vi "ObtenerDatosdelatabla.vi"(7 "tipo_gen":string="externo", 9 "Column":i32, 10 "Row":i32, 11 "Prueba32 in":refnum<class "Prueba031.lvclass">) -> (3 "Prueba32 out":refnum<class "Prueba031.lvclass">)   [LabVIEW 2019, in "Prueba031.lvclass"]
uses:
  Prueba031.lvclass
  Prueba031.lvclass/Prueba031.ctl
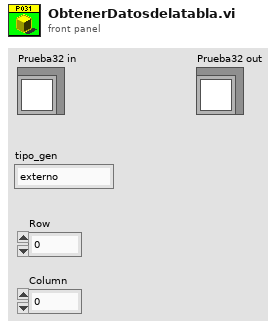
[diagram p1: front panel]
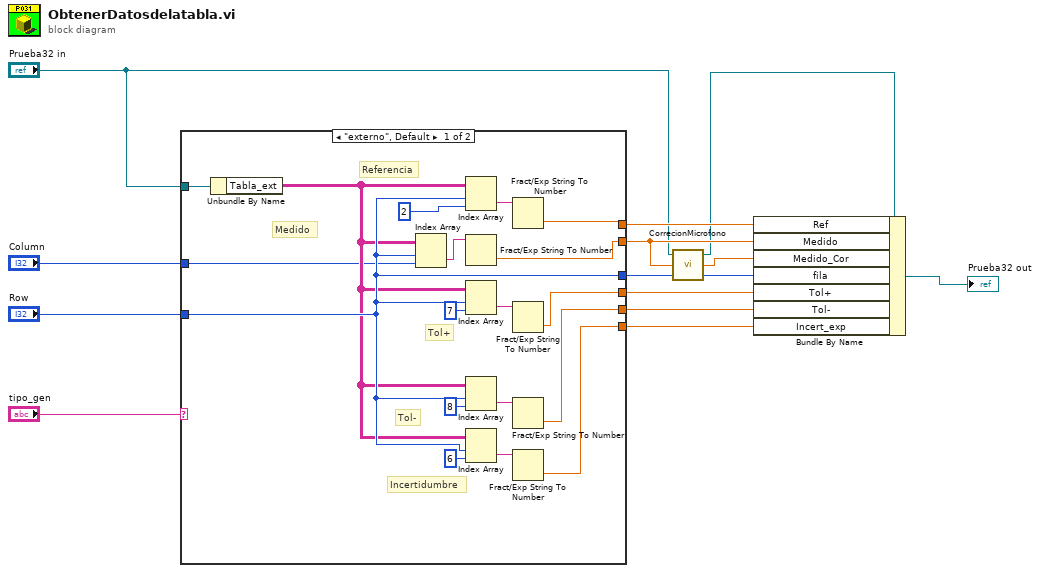
[diagram p0: block diagram]
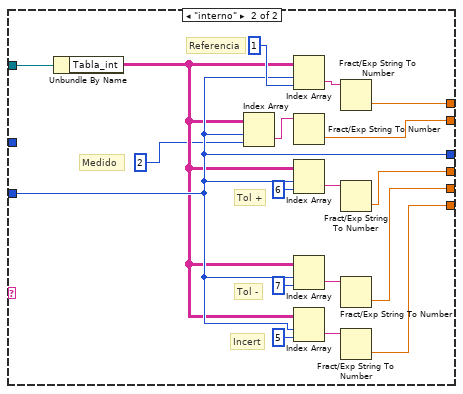
[diagram p2: hidden frame]
diagram:
  n1 = case shown="\"externo\", Default" "tipo_gen" {
    tunnel: [w32 w50] -> w14
    tunnel: "Row" -> [w20 w38]
    tunnel: [w28 w46] -> w12
    tunnel: [w25 w43] -> w11
    tunnel: "Column" -> [w15 _]
    tunnel: [w20 w38] -> w6
    tunnel: "Prueba32 in" -> [w19 w37]
    tunnel: [w17 w35] -> w7
    tunnel: [w16 w34] -> w4
    frame "externo", Default {
      # "Referencia"
      # "Tol+"
      # "Tol-"
      # "Incertidumbre"
      # "Medido"
      n2 = Unbundle By Name(w19) -> ("Tabla_ext"=w18:string[][])
      n3 = Index Array(array=w18, index (row)=w20, index (col)=w15) -> (element=w21:string)
      n4 = Index Array(array=w18, index (row)=w20, index (col)=2 ("disabled index (col)")) -> (element=w23:string)
      n5 = Fract/Exp String To Number(string=w21) -> (number=w16:dbl)  [unwired: 3 in, 1 out]
      n6 = Index Array(array=w18, index (row)=w20, index (col)=7 ("disabled index (col)")) -> (element=w24:string)
      n7 = Index Array(array=w18, index (row)=w20, index (col)=8 ("disabled index (col)")) -> (element=w27:string)
      n8 = Index Array(array=w18, index (row)=w20, index (col)=6 ("disabled index (col)")) -> (element=w31:string)
      n9 = Fract/Exp String To Number(string=w23) -> (number=w17:dbl)  [unwired: 3 in, 1 out]
      n10 = Fract/Exp String To Number(string=w24) -> (number=w25:dbl)  [unwired: 3 in, 1 out]
      n11 = Fract/Exp String To Number(string=w27) -> (number=w28:dbl)  [unwired: 3 in, 1 out]
      n12 = Fract/Exp String To Number(string=w31) -> (number=w32:dbl)  [unwired: 3 in, 1 out]
    }
    frame "interno" {
      # "Referencia"
      # "Medido"
      # "Incert"
      # "Tol -"
      # "Tol +"
      n13 = Unbundle By Name(w37) -> ("Tabla_int"=w36:string[][])
      n14 = Index Array(array=w36, index (row)=w38, index (col)=2 ("disabled index (col)")) -> (element=w39:string)
      n15 = Index Array(array=w36, index (row)=w38, index (col)=1 ("disabled index (col)")) -> (element=w41:string)
      n16 = Fract/Exp String To Number(string=w39) -> (number=w34:dbl)  [unwired: 3 in, 1 out]
      n17 = Index Array(array=w36, index (row)=w38, index (col)=6 ("disabled index (col)")) -> (element=w42:string)
      n18 = Index Array(array=w36, index (row)=w38, index (col)=7 ("disabled index (col)")) -> (element=w45:string)
      n19 = Index Array(array=w36, index (row)=w38, index (col)=5 ("disabled index (col)")) -> (element=w49:string)
      n20 = Fract/Exp String To Number(string=w41) -> (number=w35:dbl)  [unwired: 3 in, 1 out]
      n21 = Fract/Exp String To Number(string=w42) -> (number=w43:dbl)  [unwired: 3 in, 1 out]
      n22 = Fract/Exp String To Number(string=w45) -> (number=w46:dbl)  [unwired: 3 in, 1 out]
      n23 = Fract/Exp String To Number(string=w49) -> (number=w50:dbl)  [unwired: 3 in, 1 out]
    }
  }
  n24 = call "CorrecionMicrofono.vi"("row in"=w6, "Medido"=w4, "Prueba031 in"="Prueba32 in") -> ("row out"=w5:i32, "Medido Corregido"=w1:dbl, "Prueba031 out"=w2:refnum<class "Prueba031.lvclass">)
  n25 = Bundle By Name(cluster=w2, "Ref"=w7, "Medido"=w4, "Medido_Cor"=w1, "fila"=w5, "Tol+"=w11, "Tol-"=w12, "Incert_exp"=w14) -> (→"Prueba32 out":refnum<class "Prueba031.lvclass">)
